vi "Perform Action.vi"(8 "error in":errorcluster, 10 "Input":variant, 11 "HSU MCU V2 in":refnum<class "HSU MCU V2 CFG Simulated.lvclass">) -> (0 "error out":errorcluster, 2 "Output":variant, 3 "HSU MCU V2 out":refnum<class "HSU MCU V2 CFG Simulated.lvclass">)   [LabVIEW 2024, in "HSU MCU V2 CFG Simulated.lvclass"]
uses:
  HSU MCU V2 CFG Simulated.lvclass
  HSU MCU V2 CFG/HSU MCU V2 CFG.lvclass
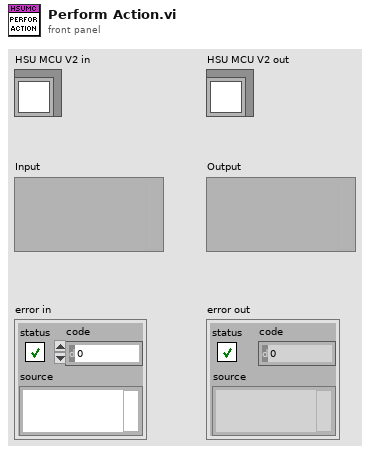
[diagram p1: front panel]
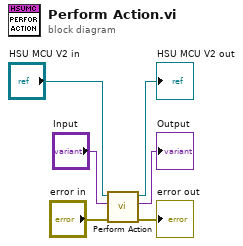
[diagram p0: block diagram]
diagram:
  n1 = call-parent "Perform Action.vi"("error in"="error in", "Input"="Input", "HSU MCU V2 in"="HSU MCU V2 in") -> ("error out"=→"error out":errorcluster, "Output"=→"Output":variant, "HSU MCU V2 out"=→"HSU MCU V2 out":refnum<class "HSU MCU V2 CFG Simulated.lvclass">)  [unwired: 6 in]
